vi "Analog_Input_4Channels_W24I5.vi"(1 "IO":T1={"AI 0"="Mod2/AI0", "AI 1"="Mod2/AI0", "AI 2"="Mod2/AI0", "AI 3"="Mod2/AI0"}) -> (0 "Values":fxp<+/-,24,5>[](array[numeric]))   [LabVIEW 2019, in "FPGA Wizard Templates.lvlib"]
uses:
  FPGA Wizard Templates.lvlib
  <vilib>/eio/EIONode/EIONode.xnode
  <vilib>/rvi/eio/common/nirviEmuTemplateMethod_errors.vi
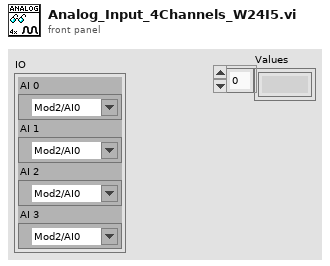
[diagram p1: front panel]
types:
  T1 = cluster{"AI 0":refnum<k21>, "AI 1":refnum<k21>, "AI 2":refnum<k21>, "AI 3":refnum<k21>}
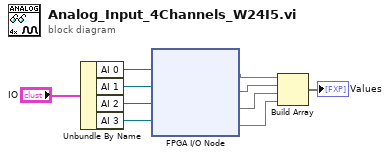
[diagram p0: block diagram]
diagram:
  n1 = Unbundle By Name("IO") -> ("AI 0"=w9:refnum<k21>, "AI 1"=w8:refnum<k21>, "AI 2"=w7:refnum<k21>, "AI 3"=w6:refnum<k21>)
  n2 = xnode "FPGA I/O Node"("FPGA I/O In"=w9, "FPGA I/O In"=w8, "FPGA I/O In"=w7, "FPGA I/O In"=w6) -> ("I/O Item"=w5, "I/O Item"=w4, "I/O Item"=w3, "I/O Item"=w2)  [unwired: 4 out]
  n3 = Build Array(w5, w4, w3, w2) -> (→"Values":void[])
